vi "I2C Utility.vi"(0 "Handle In":i32, 1 "I2C_SDA_DIONUM":i32=-1, 2 "I2C_SCL_DIONUM":i32=-1, 5 "I2C_SPEED_THROTTLE":i32=-1, 7 "I2C_OPTIONS":i32=-1, 9 "I2C_SLAVE_ADDRESS":i32=-1, 11 "error in":errorcluster, 12 "I2C_NUM_BYTES_RX":i32=-1, 13 "I2C_WRITE_DATA":i32[](array[numeric])) -> (4 "Handle Out":i32, 6 "Data Read":dbl[](array[numeric]), 10 "Acks Received":dbl, 14 "I2C COM Error Out":errorcluster, 15 "error out":errorcluster)   [LabVIEW 2020]
panel:
  out "Directions":i32[](array[numeric])
  out "numValues":i32[](array[numeric])
  out "Values":dbl[][](array[numeric])
  out "Names":string[](array[string])
  out "ErrorAddress":i32
  out "Results":dbl[][](array[numeric]) format="%.2f"
  # "Input & Output Variables:"
  # "Open LabJack Device Handle"
  # "Return LabJack Device Handle"
  # "-1: Not Configured\nval >-1: Config I2C_SDA_DIONUM"
  # "Acks Received: Binary Array"
  # "-1: Not Configured\nval >-1: Config I2C_SCL_DIONUM"
  # "Data Read by device"
  # "-1: Not Configured\nval >-1: Config I2C_SPEED_THROTTLE"
  # "-1: Not Configured\nval >-1: Config I2C_OPTIONS"
  # "-1: Not Configured\nval >-1: Config I2C_SLAVE_ADDRESS"
  # "-1: Not Configured\nval >-1: Config I2C_NUM_BYTES_RX"
  # "If: Acks Received == 0, report Error\nElse: Report No Error"
  # "All Array Lengths: Configure I2C_NUM_BYTES_TX\nArray Lengths >0: Write I2C_WRITE_DATA"
  # "Return LJM Error"
  # "Values Sent & Received from the LJM_eNames Function Call:"
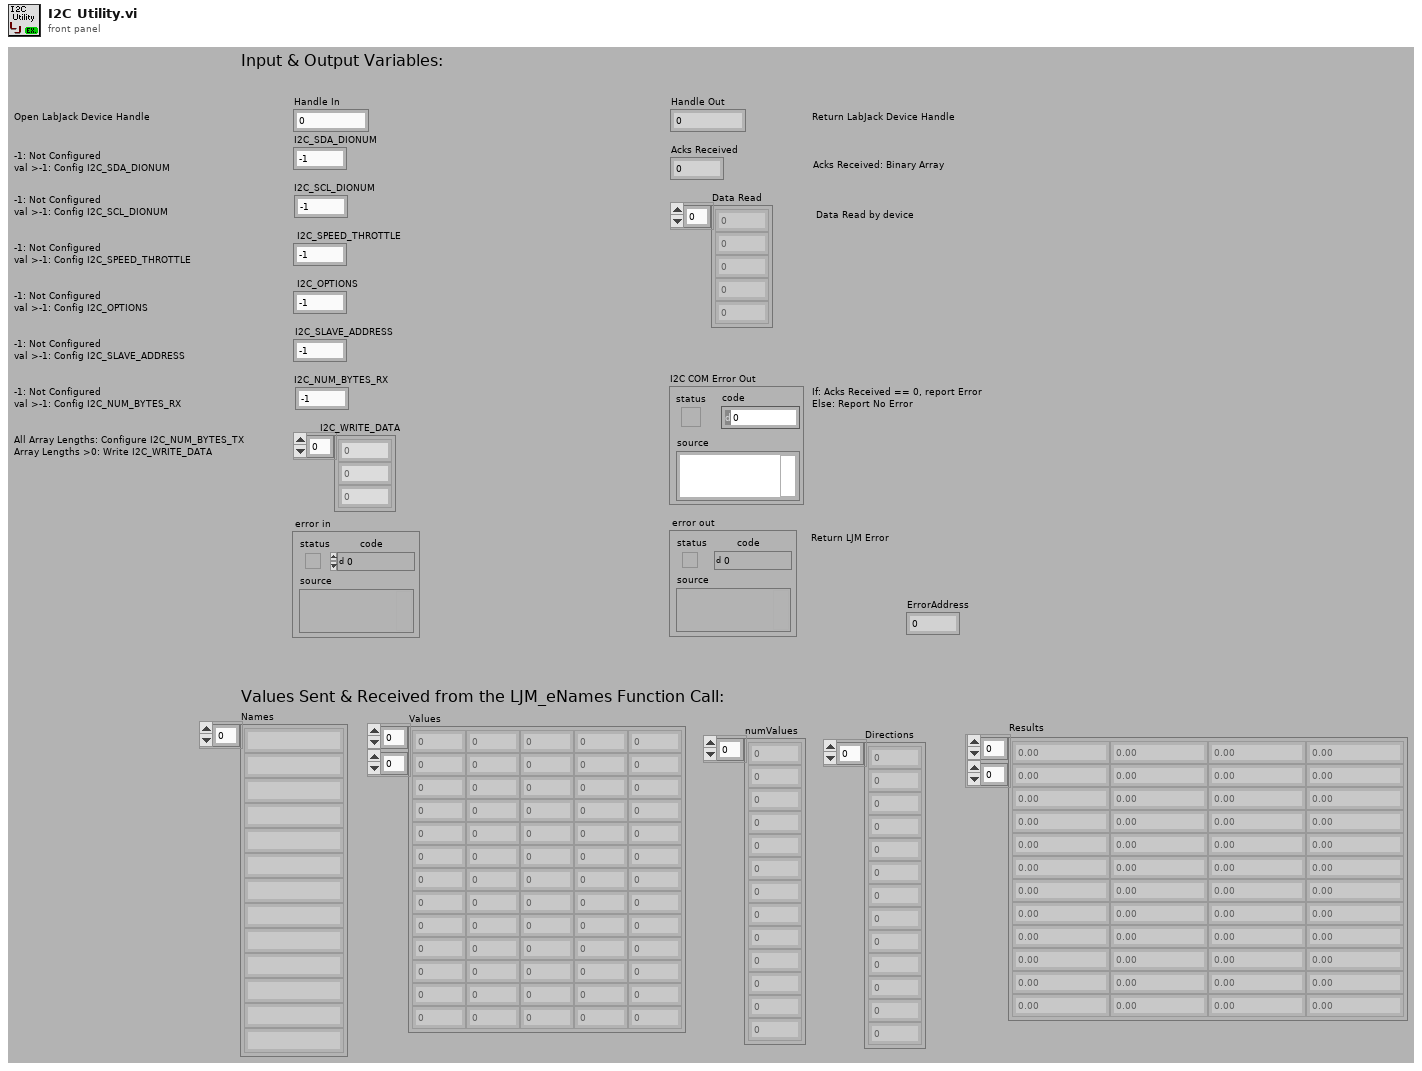
[diagram p1: front panel]
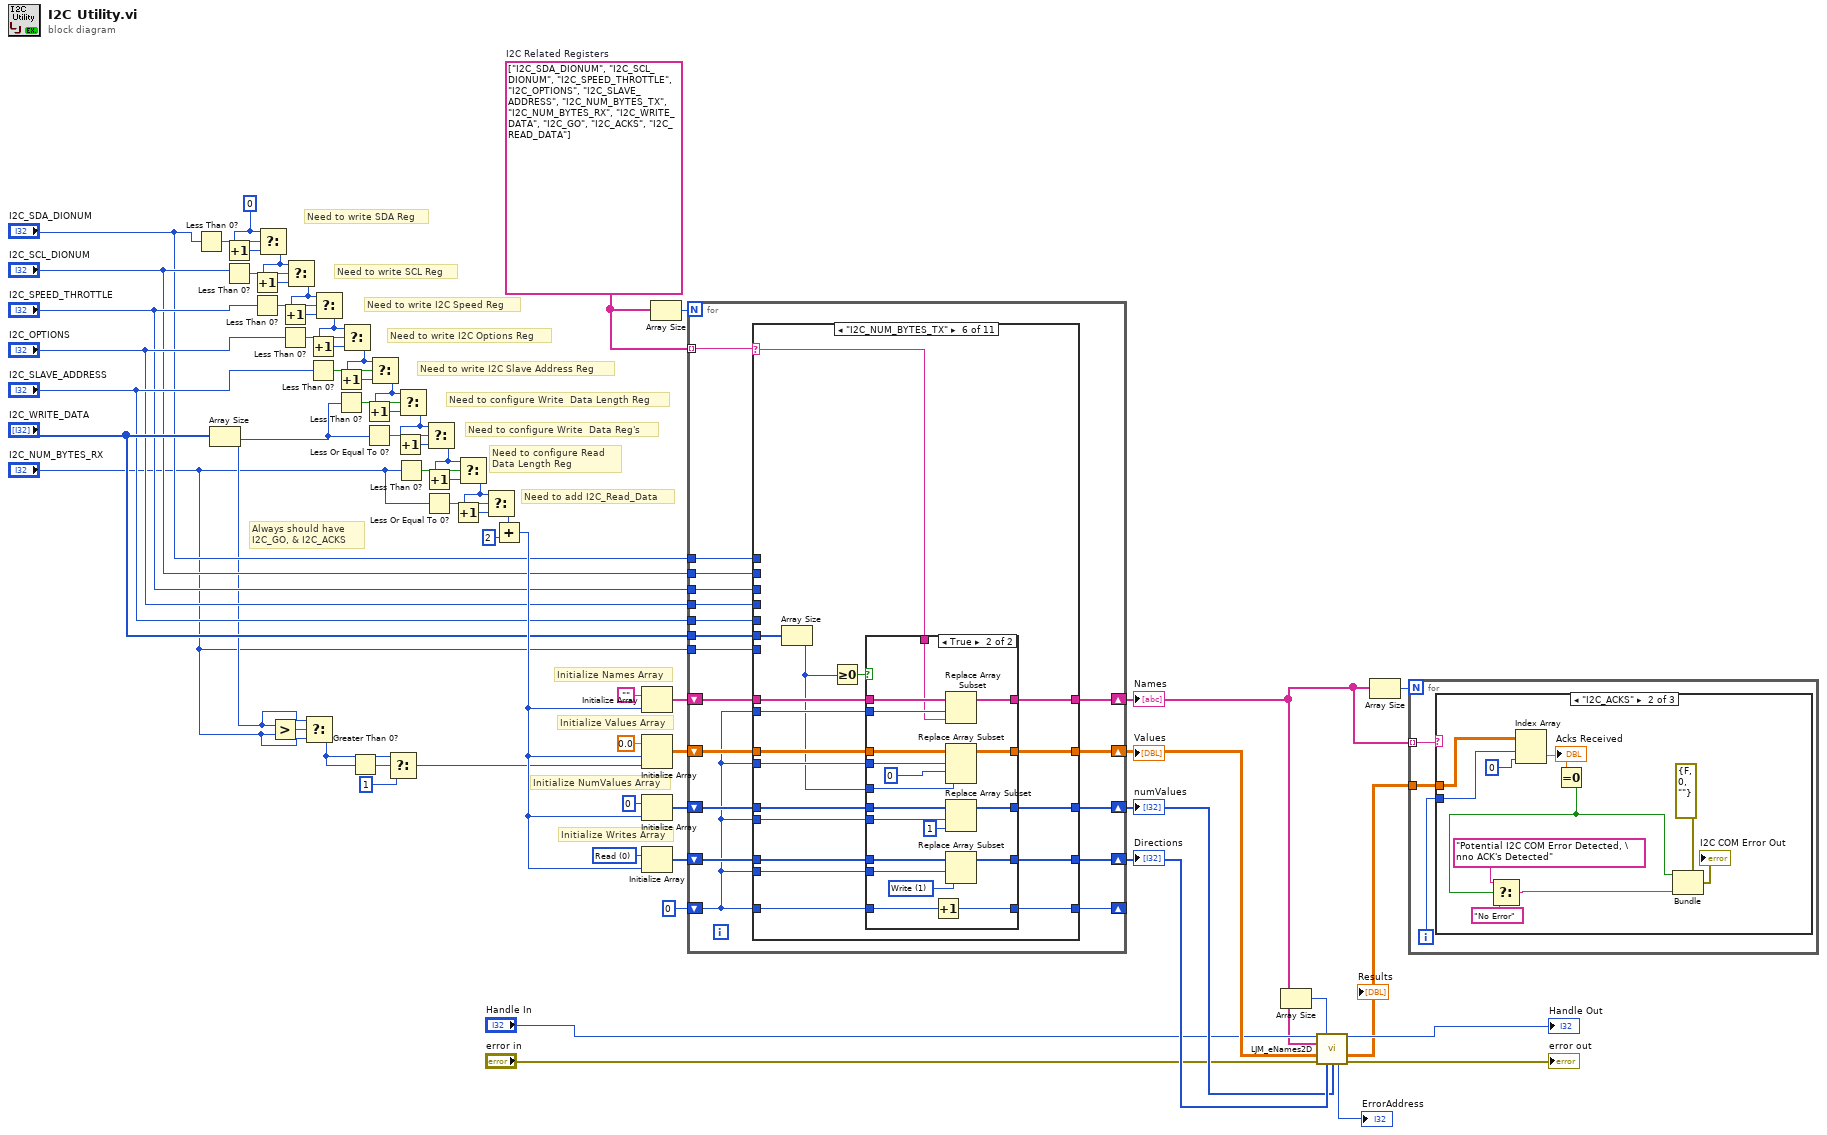
[diagram p0: block diagram]
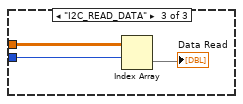
[diagram p3: hidden frame]
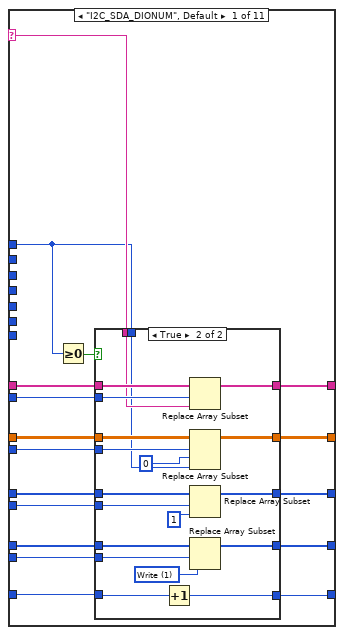
[diagram p4: hidden frame]
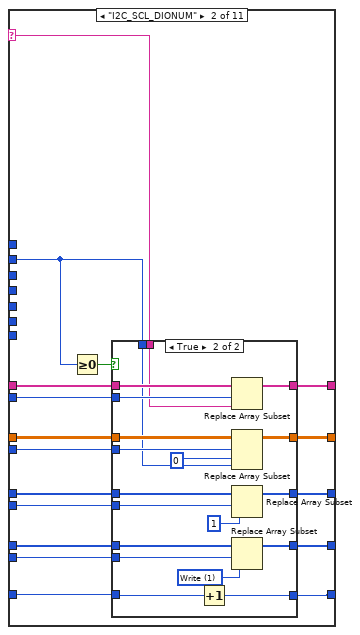
[diagram p6: hidden frame]
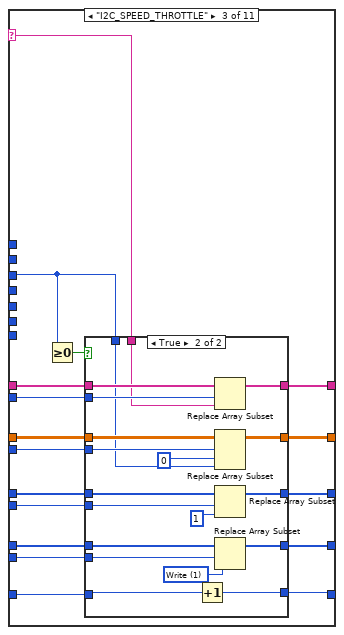
[diagram p8: hidden frame]
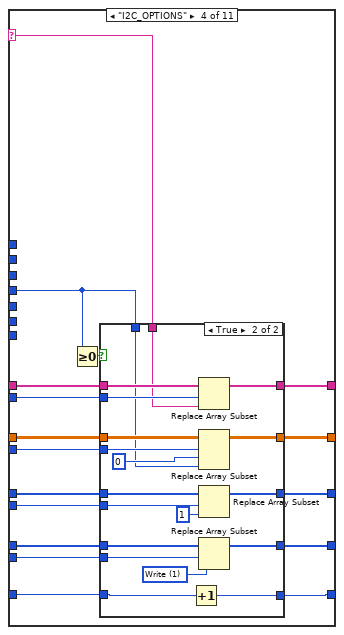
[diagram p10: hidden frame]
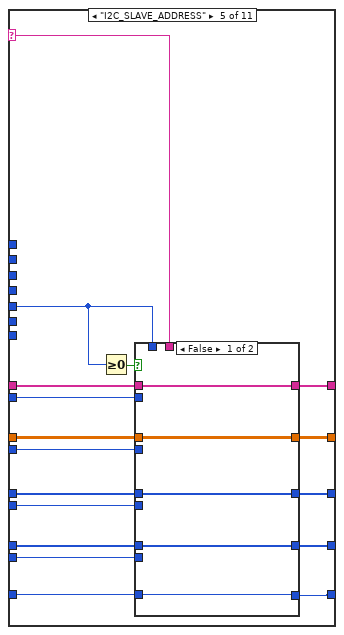
[diagram p12: hidden frame]
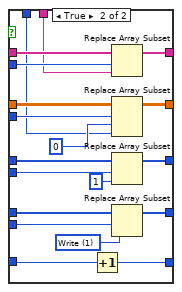
[diagram p13: hidden frame]
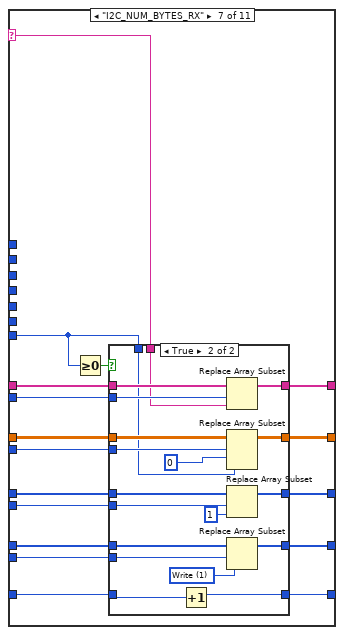
[diagram p15: hidden frame]
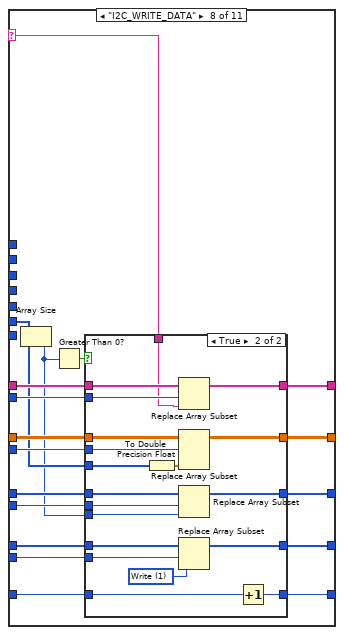
[diagram p17: hidden frame]
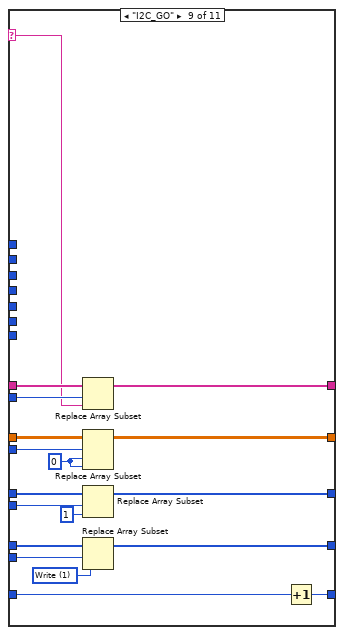
[diagram p19: hidden frame]
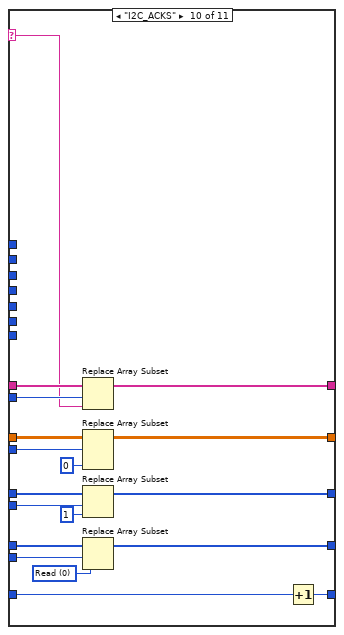
[diagram p20: hidden frame]
diagram:
  w41 = 0 items=["Read", "Write"] ("Ring")
  w34 = string[] ["I2C_SDA_DIONUM", "I2C_SCL_DIONUM", "I2C_SPEED_THROTTLE", "I2C_OPTIONS", "I2C_SLAVE_ADDRESS", "I2C_NUM_BYTES_TX", "I2C_NUM_BYTES_RX", "I2C_WRITE_DATA", "I2C_GO", "I2C_ACKS", "I2C_READ_DATA"]  # I2C Related Registers
  w64 = 0
  # "Need to add I2C_Read_Data"
  # "Need to configure Write  Data Reg's"
  # "Initialize Writes Array"
  # "Initialize NumValues Array"
  # "Initialize Values Array"
  # "Initialize Names Array"
  # "Always should have\nI2C_GO, & I2C_ACKS"
  # "Need to configure Read \nData Length Reg"
  # "Need to configure Write  Data Length Reg"
  # "Need to write I2C Slave Address Reg"
  # "Need to write I2C Options Reg"
  # "Need to write I2C Speed Reg"
  # "Need to write SCL Reg"
  # "Need to write SDA Reg"
  n1 = Less Than 0?(x="I2C_SDA_DIONUM") -> (x < 0?=w65:bool)
  n2 = Array Size(array="I2C_WRITE_DATA") -> (size(s)=w26:i32)
  n3 = Increment(x=w64) -> (x+1=w66:i32)
  n4 = Less Than 0?(x="I2C_SCL_DIONUM") -> (x < 0?=w62:bool)
  n5 = Less Than 0?(x="I2C_SPEED_THROTTLE") -> (x < 0?=w59:bool)
  n6 = Select(t=w64, s=w65, f=w66) -> (s? t:f=w61:i32)
  n7 = Increment(x=w61) -> (x+1=w63:i32)
  n8 = Greater?(x=w26, y="I2C_NUM_BYTES_RX") -> (0:w43:bool)
  n9 = Less Than 0?(x="I2C_OPTIONS") -> (x < 0?=w56:bool)
  n10 = Select(t=w61, s=w62, f=w63) -> (s? t:f=w58:i32)
  n11 = Increment(x=w58) -> (x+1=w60:i32)
  n12 = Select(t=w26, s=w43, f="I2C_NUM_BYTES_RX") -> (s? t:f=w15:i32)
  n13 = Less Than 0?(x="I2C_SLAVE_ADDRESS") -> (x < 0?=w53:bool)
  n14 = Select(t=w58, s=w59, f=w60) -> (s? t:f=w55:i32)
  n15 = Increment(x=w55) -> (x+1=w57:i32)
  n16 = Less Than 0?(x=w26) -> (x < 0?=w51:bool)
  n17 = Select(t=w55, s=w56, f=w57) -> (s? t:f=w52:i32)
  n18 = Increment(x=w52) -> (x+1=w54:i32)
  n19 = Greater Than 0?(x=w15) -> (x > 0?=w16:bool)
  n20 = Less Or Equal To 0?(x=w26) -> (x <= 0?=w27:bool)
  n21 = Select(t=w52, s=w53, f=w54) -> (s? t:f=w46:i32)
  n22 = Increment(x=w46) -> (x+1=w47:i32)
  n23 = Select(t=w15, s=w16, f=1) -> (s? t:f=w13:i32)
  n24 = Less Than 0?(x="I2C_NUM_BYTES_RX") -> (x < 0?=w50:bool)
  n25 = Select(t=w46, s=w51, f=w47) -> (s? t:f=w20:i32)
  n26 = Increment(x=w20) -> (x+1=w21:i32)
  n27 = Less Or Equal To 0?(x="I2C_NUM_BYTES_RX") -> (x <= 0?=w25:bool)
  n28 = Select(t=w20, s=w27, f=w21) -> (s? t:f=w24:i32)
  n29 = Increment(x=w24) -> (x+1=w48:i32)
  n30 = Select(t=w24, s=w50, f=w48) -> (s? t:f=w18:i32)
  n31 = Increment(x=w18) -> (x+1=w19:i32)
  n32 = Select(t=w18, s=w25, f=w19) -> (s? t:f=w22:i32)
  n33 = Add(x=w22, y=2) -> (x+y=w40:i32)
  n34 = Initialize Array("", w40) -> (w38:string[])
  n35 = Initialize Array(0.0 ("element"), w40, w13) -> (w37:dbl[][])
  n36 = Initialize Array(0, w40) -> (w36:i32[])
  n37 = Initialize Array(w41, w40) -> (w35:i32[])
  n38 = Array Size(array=w34) -> (size(s)=w44:i32)
  n39 = for {
    N: w44 -> [_]
    tunnel: w34 -> [w84] mode=indexing
    shift-right: [w72] -> w1
    shift-left: w38 -> [w76]
    shift-right: [w71] -> w12
    shift-left: w37 -> [w75]
    shift-right: [w70] -> w10
    shift-left: w36 -> [w74]
    shift-right: [w69] -> w11
    shift-left: w35 -> [w73]
    tunnel: "I2C_NUM_BYTES_RX" -> [w83]
    tunnel: "I2C_WRITE_DATA" -> [w82]
    tunnel: "I2C_SLAVE_ADDRESS" -> [w81]
    tunnel: "I2C_OPTIONS" -> [w80]
    tunnel: "I2C_SPEED_THROTTLE" -> [w79]
    tunnel: "I2C_SCL_DIONUM" -> [w78]
    tunnel: "I2C_SDA_DIONUM" -> [w77]
    shift-right: [w68] -> _
    shift-left: 0 -> [w67]
    n40 = case shown="\"I2C_NUM_BYTES_TX\"" w84 {
      selector: w84 -> [w89 w130 w171 w212 w253 w295 w336 w378 w420 w438 w455]
      tunnel: w83 -> [_ _ _ _ _ _ w334 _ _ _ w453]
      tunnel: w82 -> [_ _ _ _ _ w294 _ w377 _ _ _]
      tunnel: w81 -> [_ _ _ _ w251 _ _ _ _ _ _]
      tunnel: w80 -> [_ _ _ w210 _ _ _ _ _ _ _]
      tunnel: w79 -> [_ _ w170 _ _ _ _ _ _ _ _]
      tunnel: w78 -> [_ w128 _ _ _ _ _ _ _ _ _]
      tunnel: w77 -> [w87 _ _ _ _ _ _ _ _ _ _]
      tunnel: w76 -> [w101 w142 w183 w224 w265 w307 w348 w390 w432 w450 w467]
      tunnel: w75 -> [w96 w141 w181 w222 w263 w305 w346 w388 w430 w448 w463]
      tunnel: w74 -> [w94 w139 w179 w220 w261 w303 w344 w386 w428 w446 w464]
      tunnel: w73 -> [w92 w136 w177 w218 w259 w301 w342 w384 w426 w444 w465]
      tunnel: [w99 w134 w175 w216 w257 w299 w340 w382 w424 w442 w462] -> w72
      tunnel: [w98 w133 w174 w215 w256 w298 w339 w381 w423 w441 w461] -> w71
      tunnel: [w97 w132 w173 w214 w255 w297 w338 w380 w422 w440 w460] -> w70
      tunnel: [w90 w131 w172 w213 w254 w296 w337 w379 w421 w439 w459] -> w69
      tunnel: w67 -> [w100 w140 w182 w223 w264 w306 w347 w389 w431 w449 w466]
      tunnel: w67 -> [w93 w137 w178 w219 w260 w302 w343 w385 w427 w445 w458]
      tunnel: w67 -> [w91 w135 w176 w217 w258 w300 w341 w383 w425 w443 w457]
      tunnel: w67 -> [w95 w138 w180 w221 w262 w304 w345 w387 w429 w447 w456]
      tunnel: w67 -> [w86 w127 w168 w209 w250 w291 w333 w374 w415 w433 w451]
      tunnel: [w85 w126 w167 w208 w249 w290 w332 w373 w416 w434 w452] -> w68
      frame "I2C_SDA_DIONUM", Default {
        n41 = Greater Or Equal To 0?(x=w87) -> (x >= 0?=w88:bool)
        n42 = case shown="True" w88 {
          tunnel: w101 -> [w106 w125]
          tunnel: w100 -> [_ w124]
          tunnel: [w106 w123] -> w99
          tunnel: [w105 w122] -> w98
          tunnel: [w104 w121] -> w97
          tunnel: w96 -> [w105 w120]
          tunnel: w95 -> [_ w119]
          tunnel: w94 -> [w104 w118]
          tunnel: w93 -> [_ w117]
          tunnel: w92 -> [w103 w116]
          tunnel: w91 -> [_ w115]
          tunnel: [w103 w114] -> w90
          tunnel: w89 -> [_ w113]
          tunnel: w87 -> [_ w112]
          tunnel: w86 -> [w102 w108]
          tunnel: [w102 w107] -> w85
          frame False {
          }
          frame True {
            w110 = 1 items=["Read", "Write"] ("Ring")
            n43 = Increment(x=w108) -> (x+1=w107:i32)
            n44 = Replace Array Subset(array=w125, new element=w113, index=w124) -> (w123:string[])
            n45 = Replace Array Subset(array=w120, new element=w112, index (row)=w119, index (col)=0 ("disabled index (col)")) -> (w122:dbl[][])
            n46 = Replace Array Subset(array=w118, new element=1, index=w117) -> (w121:i32[])
            n47 = Replace Array Subset(array=w116, new element=w110, index=w115) -> (w114:i32[])
          }
        }
      }
      frame "I2C_SCL_DIONUM" {
        n48 = Greater Or Equal To 0?(x=w128) -> (x >= 0?=w129:bool)
        n49 = case shown="True" w129 {
          tunnel: w142 -> [w147 w166]
          tunnel: w141 -> [w146 w165]
          tunnel: w140 -> [_ w164]
          tunnel: w139 -> [w145 w163]
          tunnel: w138 -> [_ w162]
          tunnel: w137 -> [_ w161]
          tunnel: w136 -> [w144 w160]
          tunnel: w135 -> [_ w159]
          tunnel: [w147 w158] -> w134
          tunnel: [w146 w157] -> w133
          tunnel: [w145 w156] -> w132
          tunnel: [w144 w155] -> w131
          tunnel: w130 -> [_ w154]
          tunnel: w128 -> [_ w152]
          tunnel: w127 -> [w143 w149]
          tunnel: [w143 w148] -> w126
          frame False {
          }
          frame True {
            w150 = 1 items=["Read", "Write"] ("Ring")
            n50 = Increment(x=w149) -> (x+1=w148:i32)
            n51 = Replace Array Subset(array=w166, new element=w154, index=w164) -> (w158:string[])
            n52 = Replace Array Subset(array=w165, new element=w152, index (row)=w162, index (col)=0) -> (w157:dbl[][])
            n53 = Replace Array Subset(array=w163, new element=1, index=w161) -> (w156:i32[])
            n54 = Replace Array Subset(array=w160, new element=w150, index=w159) -> (w155:i32[])
          }
        }
      }
      frame "I2C_SPEED_THROTTLE" {
        n55 = Greater Or Equal To 0?(x=w170) -> (x >= 0?=w169:bool)
        n56 = case shown="True" w169 {
          tunnel: w183 -> [w188 w207]
          tunnel: w182 -> [_ w206]
          tunnel: w181 -> [w187 w205]
          tunnel: w180 -> [_ w204]
          tunnel: w179 -> [w186 w203]
          tunnel: w178 -> [_ w202]
          tunnel: w177 -> [w185 w201]
          tunnel: w176 -> [_ w200]
          tunnel: [w188 w199] -> w175
          tunnel: [w187 w198] -> w174
          tunnel: [w186 w197] -> w173
          tunnel: [w185 w196] -> w172
          tunnel: w171 -> [_ w195]
          tunnel: w170 -> [_ w193]
          tunnel: w168 -> [w184 w190]
          tunnel: [w184 w189] -> w167
          frame False {
          }
          frame True {
            w191 = 1 items=["Read", "Write"] ("Ring")
            n57 = Increment(x=w190) -> (x+1=w189:i32)
            n58 = Replace Array Subset(array=w207, new element=w195, index=w206) -> (w199:string[])
            n59 = Replace Array Subset(array=w205, new element=w193, index (row)=w204, index (col)=0) -> (w198:dbl[][])
            n60 = Replace Array Subset(array=w203, new element=1, index=w202) -> (w197:i32[])
            n61 = Replace Array Subset(array=w201, new element=w191, index=w200) -> (w196:i32[])
          }
        }
      }
      frame "I2C_OPTIONS" {
        n62 = Greater Or Equal To 0?(x=w210) -> (x >= 0?=w211:bool)
        n63 = case shown="True" w211 {
          tunnel: w224 -> [w229 w248]
          tunnel: w223 -> [_ w247]
          tunnel: w222 -> [w228 w246]
          tunnel: w221 -> [_ w245]
          tunnel: w220 -> [w227 w244]
          tunnel: w219 -> [_ w243]
          tunnel: w218 -> [w226 w242]
          tunnel: w217 -> [_ w241]
          tunnel: [w229 w240] -> w216
          tunnel: [w228 w239] -> w215
          tunnel: [w227 w238] -> w214
          tunnel: [w226 w237] -> w213
          tunnel: w212 -> [_ w236]
          tunnel: w210 -> [_ w234]
          tunnel: w209 -> [w225 w231]
          tunnel: [w225 w230] -> w208
          frame False {
          }
          frame True {
            w232 = 1 items=["Read", "Write"] ("Ring")
            n64 = Increment(x=w231) -> (x+1=w230:i32)
            n65 = Replace Array Subset(array=w248, new element=w236, index=w247) -> (w240:string[])
            n66 = Replace Array Subset(array=w246, new element=w234, index (row)=w245, index (col)=0 ("disabled index (col)")) -> (w239:dbl[][])
            n67 = Replace Array Subset(array=w244, new element=1 ("new element/subarray"), index=w243) -> (w238:i32[])
            n68 = Replace Array Subset(array=w242, new element=w232, index=w241) -> (w237:i32[])
          }
        }
      }
      frame "I2C_SLAVE_ADDRESS" {
        n69 = Greater Or Equal To 0?(x=w251) -> (x >= 0?=w252:bool)
        n70 = case shown="False" w252 {
          tunnel: w265 -> [w270 w289]
          tunnel: w264 -> [_ w288]
          tunnel: w263 -> [w269 w287]
          tunnel: w262 -> [_ w286]
          tunnel: w261 -> [w268 w285]
          tunnel: w260 -> [_ w284]
          tunnel: w259 -> [w267 w283]
          tunnel: w258 -> [_ w282]
          tunnel: [w270 w281] -> w257
          tunnel: [w269 w280] -> w256
          tunnel: [w268 w279] -> w255
          tunnel: [w267 w278] -> w254
          tunnel: w253 -> [_ w277]
          tunnel: w251 -> [_ w275]
          tunnel: w250 -> [w266 w272]
          tunnel: [w266 w271] -> w249
          frame False {
          }
          frame True {
            w273 = 1 items=["Read", "Write"] ("Ring")
            n71 = Increment(x=w272) -> (x+1=w271:i32)
            n72 = Replace Array Subset(array=w289, new element=w277, index=w288) -> (w281:string[])
            n73 = Replace Array Subset(array=w287, new element=w275, index (row)=w286, index (col)=0 ("disabled index (col)")) -> (w280:dbl[][])
            n74 = Replace Array Subset(array=w285, new element=1 ("new element/subarray"), index=w284) -> (w279:i32[])
            n75 = Replace Array Subset(array=w283, new element=w273, index=w282) -> (w278:i32[])
          }
        }
      }
      frame "I2C_NUM_BYTES_TX" {
        n76 = Array Size(array=w294) -> (size(s)=w292:i32)
        n77 = Greater Or Equal To 0?(x=w292) -> (x >= 0?=w293:bool)
        n78 = case shown="True" w293 {
          tunnel: w307 -> [w312 w331]
          tunnel: w306 -> [_ w330]
          tunnel: w305 -> [w311 w329]
          tunnel: w304 -> [_ w328]
          tunnel: w303 -> [w310 w327]
          tunnel: w302 -> [_ w326]
          tunnel: w301 -> [w309 w325]
          tunnel: w300 -> [_ w324]
          tunnel: [w312 w323] -> w299
          tunnel: [w311 w322] -> w298
          tunnel: [w310 w321] -> w297
          tunnel: [w309 w320] -> w296
          tunnel: w295 -> [_ w319]
          tunnel: w292 -> [_ w318]
          tunnel: w291 -> [w308 w313]
          tunnel: [w308 w314] -> w290
          frame False {
          }
          frame True {
            w315 = 1 items=["Read", "Write"] ("Ring")
            n79 = Increment(x=w313) -> (x+1=w314:i32)
            n80 = Replace Array Subset(array=w331, new element=w319, index=w330) -> (w323:string[])
            n81 = Replace Array Subset(array=w329, new element=w318, index (row)=w328, index (col)=0 ("disabled index (col)")) -> (w322:dbl[][])
            n82 = Replace Array Subset(array=w327, new element=1 ("new element/subarray"), index=w326) -> (w321:i32[])
            n83 = Replace Array Subset(array=w325, new element=w315, index=w324) -> (w320:i32[])
          }
        }
      }
      frame "I2C_NUM_BYTES_RX" {
        n84 = Greater Or Equal To 0?(x=w334) -> (x >= 0?=w335:bool)
        n85 = case shown="True" w335 {
          tunnel: w348 -> [w353 w372]
          tunnel: w347 -> [_ w371]
          tunnel: w346 -> [w352 w370]
          tunnel: w345 -> [_ w369]
          tunnel: w344 -> [w351 w368]
          tunnel: w343 -> [_ w367]
          tunnel: w342 -> [w350 w366]
          tunnel: w341 -> [_ w365]
          tunnel: [w353 w364] -> w340
          tunnel: [w352 w363] -> w339
          tunnel: [w351 w362] -> w338
          tunnel: [w350 w361] -> w337
          tunnel: w336 -> [_ w360]
          tunnel: w334 -> [_ w359]
          tunnel: w333 -> [w349 w354]
          tunnel: [w349 w355] -> w332
          frame False {
          }
          frame True {
            w356 = 1 items=["Read", "Write"] ("Ring")
            n86 = Increment(x=w354) -> (x+1=w355:i32)
            n87 = Replace Array Subset(array=w372, new element=w360, index=w371) -> (w364:string[])
            n88 = Replace Array Subset(array=w370, new element=w359, index (row)=w369, index (col)=0 ("disabled index (col)")) -> (w363:dbl[][])
            n89 = Replace Array Subset(array=w368, new element=1 ("new element/subarray"), index=w367) -> (w362:i32[])
            n90 = Replace Array Subset(array=w366, new element=w356, index=w365) -> (w361:i32[])
          }
        }
      }
      frame "I2C_WRITE_DATA" {
        n91 = Array Size(array=w377) -> (size(s)=w375:i32)
        n92 = Greater Than 0?(x=w375) -> (x > 0?=w376:bool)
        n93 = case shown="True" w376 {
          tunnel: w390 -> [w395 w414]
          tunnel: w389 -> [_ w413]
          tunnel: w388 -> [w394 w412]
          tunnel: w387 -> [_ w411]
          tunnel: w386 -> [w393 w410]
          tunnel: w385 -> [_ w409]
          tunnel: w384 -> [w392 w408]
          tunnel: w383 -> [_ w407]
          tunnel: [w395 w406] -> w382
          tunnel: [w394 w405] -> w381
          tunnel: [w393 w404] -> w380
          tunnel: [w392 w403] -> w379
          tunnel: w378 -> [_ w402]
          tunnel: w377 -> [_ w399]
          tunnel: w375 -> [_ w398]
          tunnel: w374 -> [w391 w396]
          tunnel: [w391 w397] -> w373
          frame False {
          }
          frame True {
            w400 = 1 items=["Read", "Write"] ("Ring")
            n94 = To Double Precision Float(number=w399) -> (double precision float=w401:dbl[])
            n95 = Replace Array Subset(array=w414, new element=w402, index=w413) -> (w406:string[])
            n96 = Replace Array Subset(array=w412, new element=w401, index (row)=w411) -> (w405:dbl[][])  [unwired: 1 in]
            n97 = Replace Array Subset(array=w410, new element=w398, index=w409) -> (w404:i32[])
            n98 = Replace Array Subset(array=w408, new element=w400, index=w407) -> (w403:i32[])
            n99 = Increment(x=w396) -> (x+1=w397:i32)
          }
        }
      }
      frame "I2C_GO" {
        w417 = 1 items=["Read", "Write"] ("Ring")
        w419 = 0
        n100 = Replace Array Subset(array=w432, new element=w420, index=w431) -> (w424:string[])
        n101 = Replace Array Subset(array=w430, new element=w419, index (row)=w429, index (col)=w419) -> (w423:dbl[][])
        n102 = Replace Array Subset(array=w428, new element=1 ("new element/subarray"), index=w427) -> (w422:i32[])
        n103 = Replace Array Subset(array=w426, new element=w417, index=w425) -> (w421:i32[])
        n104 = Increment(x=w415) -> (x+1=w416:i32)
      }
      frame "I2C_ACKS" {
        w435 = 0 items=["Read", "Write"] ("Ring")
        w437 = 0 ("disabled index (col)")
        n105 = Replace Array Subset(array=w450, new element=w438, index=w449) -> (w442:string[])
        n106 = Replace Array Subset(array=w448, new element=w437, index (row)=w447, index (col)=w437) -> (w441:dbl[][])
        n107 = Replace Array Subset(array=w446, new element=1 ("new element/subarray"), index=w445) -> (w440:i32[])
        n108 = Replace Array Subset(array=w444, new element=w435, index=w443) -> (w439:i32[])
        n109 = Increment(x=w433) -> (x+1=w434:i32)
      }
      frame "I2C_READ_DATA" {
        n110 = Greater Than 0?(x=w453) -> (x > 0?=w454:bool)
        n111 = case shown="False" w454 {
          tunnel: w467 -> [w472 w490]
          tunnel: w466 -> [_ w489]
          tunnel: w465 -> [w469 w488]
          tunnel: w464 -> [w470 w487]
          tunnel: w463 -> [w471 w486]
          tunnel: [w472 w485] -> w462
          tunnel: [w471 w484] -> w461
          tunnel: [w470 w483] -> w460
          tunnel: [w469 w482] -> w459
          tunnel: w458 -> [_ w481]
          tunnel: w457 -> [_ w480]
          tunnel: w456 -> [_ w479]
          tunnel: w455 -> [_ w478]
          tunnel: w453 -> [_ w475]
          tunnel: [w468 w474] -> w452
          tunnel: w451 -> [w468 w473]
          frame False {
          }
          frame True {
            w476 = 0 ("disabled index (col)")
            w477 = 0 items=["Read", "Write"] ("Ring")
            n112 = Replace Array Subset(array=w490, new element=w478, index=w489) -> (w485:string[])
            n113 = Replace Array Subset(array=w486, new element=w476, index (row)=w479, index (col)=w476) -> (w484:dbl[][])
            n114 = Replace Array Subset(array=w487, new element=w475, index=w481) -> (w483:i32[])
            n115 = Replace Array Subset(array=w488, new element=w477, index=w480) -> (w482:i32[])
            n116 = Increment(x=w473) -> (x+1=w474:i32)
          }
        }
      }
    }
  }
  "Names" <- w1
  "Values" <- w12
  "numValues" <- w10
  "Directions" <- w11
  n117 = Array Size(array=w1) -> (size(s)=w9:i32)
  n118 = call "LJM_eNames2D.vi"("Handle In"="Handle In", "NumFrames (Auto-Detect)"=w9, "aNames"=w1, "aValuesIn"=w12, "error in"="error in", "aWrites"=w11, "aNumValues"=w10) -> ("Handle Out"=→"Handle Out":i32, "aValuesOut"=w2:dbl[][], "ErrorAddress"=→"ErrorAddress":i32, "error out"=→"error out":errorcluster)  [unwired: 5 in]
  "Results" <- w2
  n119 = Array Size(array=w1) -> (size(s)=w3:i32)
  n120 = for {
    N: w3 -> [_]
    tunnel: w2 -> [w491]
    tunnel: w1 -> [w493] mode=indexing
    i -> [w492]
    n121 = case shown="\"I2C_ACKS\"" w493 {
      tunnel: w492 -> [_ w502 w506]
      tunnel: w491 -> [_ w503 w505]
      frame "", Default {
      }
      frame "I2C_ACKS" {
        n122 = Index Array(array=w503, index (row)=w502, index (col)=0 ("disabled index (col)")) -> (element=w498:dbl)
        "Acks Received" <- w498
        n123 = Equal To 0?(x=w498) -> (x = 0?=w496:bool)
        n124 = Select(t="Potential I2C COM Error Detected, \nno ACK's Detected", s=w496, f="No Error") -> (s? t:f=w495:string)
        n125 = Bundle(cluster=errorcluster {"status"=FALSE, "code"=0, "source"=""} ("error in 2"), "status"=w496, "source"=w495) -> (→"I2C COM Error Out":errorcluster)  [unwired: 1 in]
      }
      frame "I2C_READ_DATA" {
        n126 = Index Array(array=w505, index (row)=w506) -> (element=→"Data Read":dbl[])  [unwired: 1 in]
      }
    }
  }
